vi "NumericToSIString.vi"(11 "Numeric":dbl) -> (3 "SI_String":string, 5 "OK":bool)   [LabVIEW 2020]
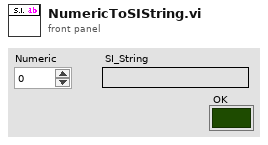
[diagram p1: front panel]
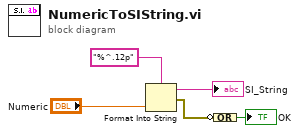
[diagram p0: block diagram]
diagram:
  n1 = Format Into String(format string="%^.12p", "Numeric") -> (resulting string=→"SI_String":string, error out=w2:errorcluster)  [unwired: 2 in]
  n2 = Compound Arithmetic op=OR(invert w2) -> (→"OK":bool)
